vi "Init Services.vi"(8 "error in (no error)":errorcluster, 11 "Vecto in":refnum<class "Vecto.lvclass">) -> (0 "error out":errorcluster, 3 "Vecto out":refnum<class "Vecto.lvclass">)   [LabVIEW 2020, in "Vecto.lvlib" / "Vecto.lvclass"]
uses:
  Vecto.lvclass
  Vecto.lvclass/Vecto.ctl
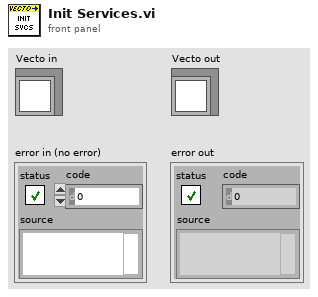
[diagram p1: front panel]
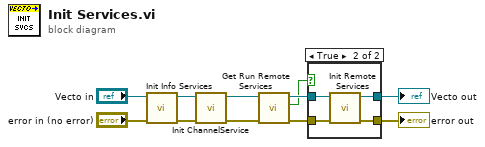
[diagram p0: block diagram]
diagram:
  n1 = call "Init Info Services.vi"("error in (no error)"="error in (no error)", "Vecto in"="Vecto in") -> ("error out"=w11:errorcluster, "Vecto out"=w10:refnum<class "Vecto.lvclass">)  [unwired: 8 in]
  n2 = call "Init ChannelService.vi"("error in (no error)"=w11, "Vecto in"=w10) -> ("error out"=w7:errorcluster, "Vecto out"=w5:refnum<class "Vecto.lvclass">)  [unwired: 8 in]
  n3 = call "Get Run Remote Services.vi"("error in (no error)"=w7, "Vecto in"=w5) -> ("error out"=w6:errorcluster, "Run Remote Services"=w3:bool, "Vecto out"=w4:refnum<class "Vecto.lvclass">)  [unwired: 7 in]
  n4 = case shown="True" w3 {
    tunnel: [w13 w15] -> w9
    tunnel: [w12 w14] -> w8
    tunnel: w4 -> [w13 w17]
    tunnel: w6 -> [w12 w16]
    frame False {
    }
    frame True {
      n5 = call "Init Remote Services.vi"("error in (no error)"=w16, "Vecto in"=w17) -> ("error out"=w14:errorcluster, "Vecto out"=w15:refnum<class "Vecto.lvclass">)  [unwired: 8 in]
    }
  }
  "error out" <- w8
  "Vecto out" <- w9
